vi "Average.vi"(8 "error in (no error)":errorcluster, 11 "XY-data":cluster{"X-array":dbl[], "Y-array":dbl[]}[](array[cluster]) {"Y-array" format="%.2p"; "X-array" format="%.2p"}) -> (0 "error out":errorcluster, 2 "Averaged XY-data out":cluster{"X-array":dbl[], "Y-array":dbl[]} {"Y-array" format="%.2p"; "X-array" format="%.2p"}, 3 "XY-data out":cluster{"X-array":dbl[], "Y-array":dbl[]}[](array[cluster]) {"Y-array" format="%.2p"; "X-array" format="%.2p"})   [LabVIEW 2019, in "xy_utilities.lvlib"]
doc: "Calculates the <b>Mean</b> of the y arrays in <b>XY-data</b> at x values defined by the <b>Configure</b> Cluster.\n\n<b>XY-data</b> is not assumed to have commensurate x values or sampling; therefore interpolation is performed before averaging.\n\nThe <b>Configure</b> cluster is used to define:\n<b>X Low</b>: Starting x value for interpolation. May lie outside of the input x array range.\n<b>X High</b>: Ending x value for interpolation. May lie outside of the input x array range.\n<b>X Step</b>: Interpolation value.\n<b>Fake Point</b>: Value added to the y array for x values outside of the x array input range.\n\nNote that this VI returns two types of data:\n<b>XY-data out</b> is the original input data array <b>XY-data</b>.\n<b>Averaged XY-data out</b> is a single containing the averaged XY-data.\n\nNote also that this is NOT a polymorphic VI. It will only work for an input that is an array of XY-data."
uses:
  xy_utilities.lvlib
  <vilib>/Analysis/NI_AALBase.lvlib
  <vilib>/Analysis/baseanly.llb/Mean (DBL).vi
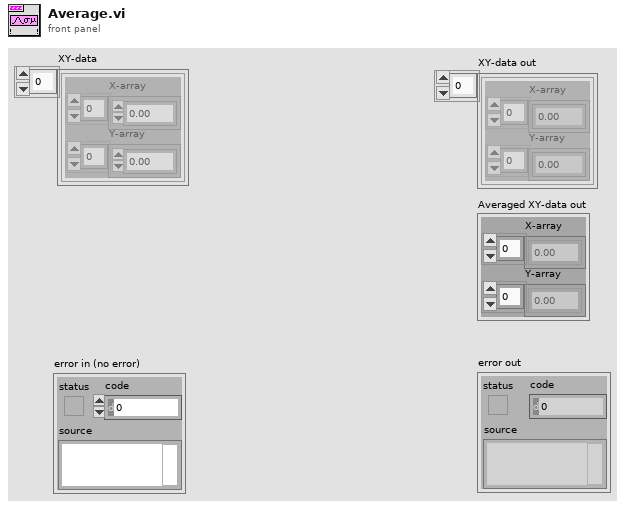
[diagram p1: front panel]
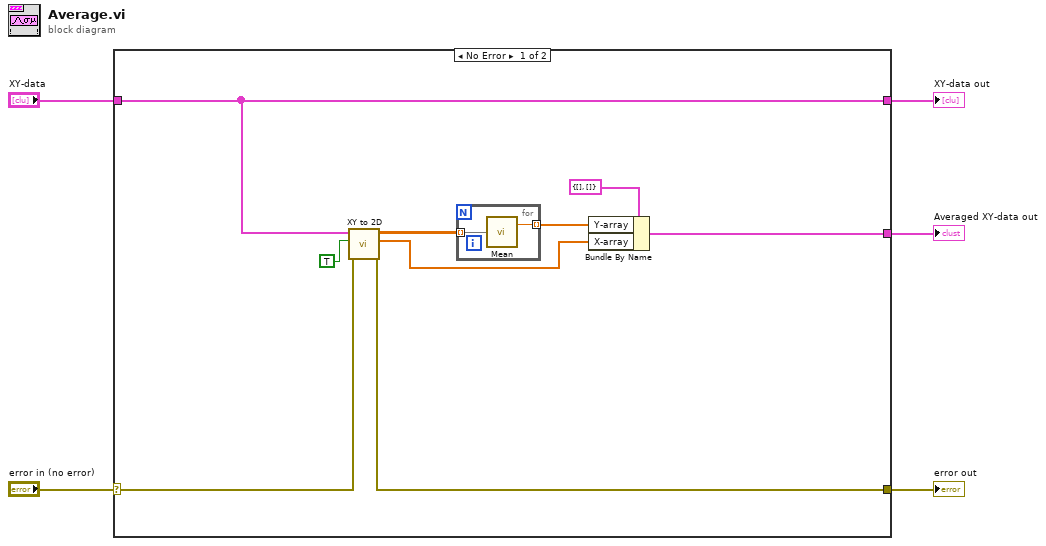
[diagram p0: block diagram]
diagram:
  n1 = case shown="No Error" "error in (no error)" {
    selector: "error in (no error)" -> [w13 w17]
    tunnel: [w11 w18] -> w5
    tunnel: "XY-data" -> [w11 w18]
    tunnel: [w12 w17] -> w4
    tunnel: [w14 _] -> w2
    frame No Error {
      n2 = call "XY to 2D.vi"("error in (no error)"=w13, "Interpolate [T]"=TRUE, "XY-data"=w11) -> ("error out"=w12:errorcluster, "X Array"=w10:dbl[], "2D Z Array"=w6:dbl[][])  [unwired: 5 in, 1 out]
      n3 = for {
        tunnel: w6 -> [w16] mode=indexing
        tunnel: [w15] -> w9 mode=indexing
        n4 = call-poly <vilib>:"Mean.vi"("X"=w16) -> ("mean"=w15:dbl)  [unwired: 1 out]
      }
      n5 = Bundle By Name(cluster=cluster{"X-array":dbl[], "Y-array":dbl[]} {"X-array"=[], "Y-array"=[]}, "Y-array"=w9, "X-array"=w10) -> (w14:cluster{"X-array":dbl[], "Y-array":dbl[]})
    }
    frame Error {
    }
  }
  "XY-data out" <- w5
  "error out" <- w4
  "Averaged XY-data out" <- w2
